vi "TW Update Supporting Projects.vi"(8 "error in (no error)":errorcluster, 10 "New Name":string, 11 "Template Project Path":path) -> (0 "error out":errorcluster)   [LabVIEW 2021, in "Plugin Generator.lvlib"]
uses:
  Plugin Generator.lvlib
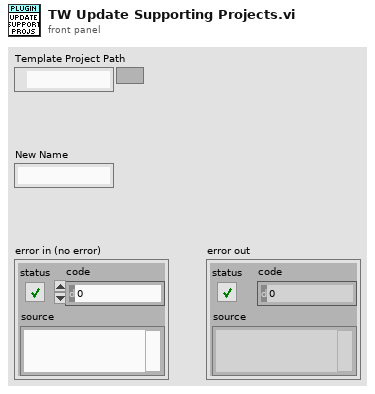
[diagram p1: front panel]
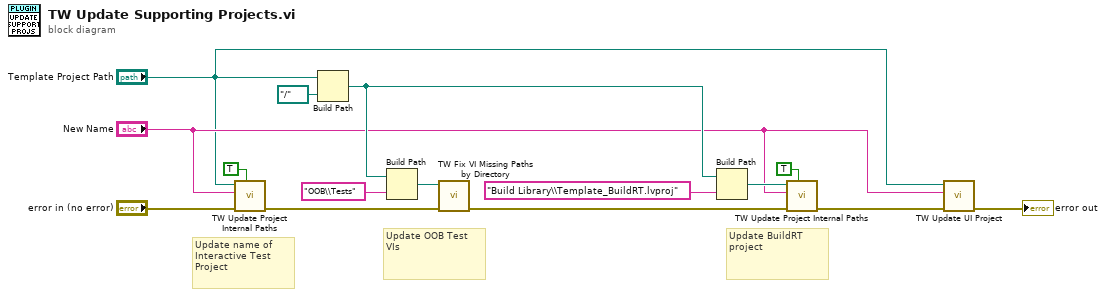
[diagram p0: block diagram]
diagram:
  # "Update BuildRT project"
  # "Update OOB Test VIs"
  # "Update name of Interactive Test Project"
  n1 = call "TW Update Project Internal Paths.vi"("Rename Project"=TRUE, "error in (no error)"="error in (no error)", "New Subname"="New Name", "Project Path"="Template Project Path") -> ("error out"=w13:errorcluster)  [unwired: 7 in]
  n2 = Build Path(base path="Template Project Path", name or relative path=path "../..") -> (appended path=w6:path)
  n3 = Build Path(base path=w6, name or relative path="OOB\\Tests" ("Class Name")) -> (appended path=w10:path)
  n4 = call "TW Fix VI Missing Paths by Directory.vi"("error in (no error)"=w13, "Folder Path"=w10) -> ("error out"=w9:errorcluster)  [unwired: 9 in]
  n5 = Build Path(base path=w6, name or relative path="Build Library\\Template_BuildRT.lvproj" ("Class Name")) -> (appended path=w8:path)
  n6 = call "TW Update Project Internal Paths.vi"("Rename Project"=TRUE, "error in (no error)"=w9, "New Subname"="New Name", "Project Path"=w8) -> ("error out"=w4:errorcluster)  [unwired: 7 in]
  n7 = call "TW Update UI Project.vi"("error in (no error)"=w4, "New Name"="New Name", "Template Project Path"="Template Project Path") -> ("error out"=→"error out":errorcluster)  [unwired: 8 in]
